vi "create tls config.vi"(8 "error in":errorcluster) -> (0 "error out":errorcluster, 3 "config out":u64)   [LabVIEW 2016, in "lv tls dll.lvlib"]
uses:
  lv tls dll.lvlib
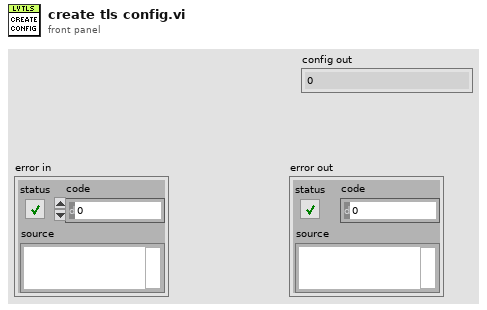
[diagram p1: front panel]
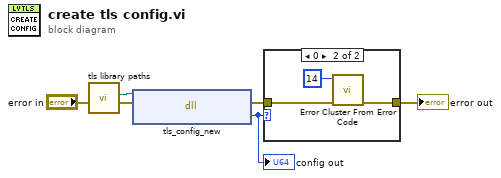
[diagram p0: block diagram]
diagram:
  n1 = call "tls library paths.vi"() -> ("libtls"=w2:path)  [unwired: 8 in, 3 out]
  n2 = dll-call lib="C:/Users/IEUser/Desktop/tlssimple/libtls-15.dll" fn="tls_config_new"(path in=w2, error in="error in") -> (error out=w4:errorcluster, "config"=w1:u64)  [unwired: 1 in, 1 out]
  "config out" <- w1
  n3 = case shown="0" w1 {
    tunnel: w4 -> [w6 w9]
    tunnel: [w6 w8] -> w5
    frame Default {
    }
    frame 0 {
      n4 = call <vilib>:"Error Cluster From Error Code.vi"("error in (no error)"=w9, "error code (0)"=14) -> ("error out"=w8:errorcluster)  [unwired: 7 in]
    }
  }
  "error out" <- w5
